vi "XY Graph Add Single Plot with Name v2.vi"(0 "XYGraph Ref in":T3, 1 "Scales (Default)":T2, 3 "Keep Existing Plots (T)":bool=TRUE, 5 "Plot":cluster{"X Array":dbl[], "Y Array":dbl[]}, 7 "Plot Metadata":variant, 9 "Plot Name (\"Plot\")":string, 11 "error in (no error)":errorcluster, 12 "Plot Style":T1) -> (4 "XY Graph Caption (or Label)":string, 8 "Plot Index":i32, 10 "Plot Name":string, 15 "error out":errorcluster)   [LabVIEW 2021, in "XY Graph Add-Ons.lvlib"]
uses:
  XY Graph Add-Ons.lvlib
  XY Graph Refnum.ctl
  Plot Scales.ctl
  Single Plot Style 2.ctl
  XY Graph Get Plots Metadata.vi
  XY Graph Get Max Legend Size.vi
  XY Graph Set Plots Metadata.vi
  Strings/Strings.lvlib
  Graphs.lvlib
  Error/Error.lvlib
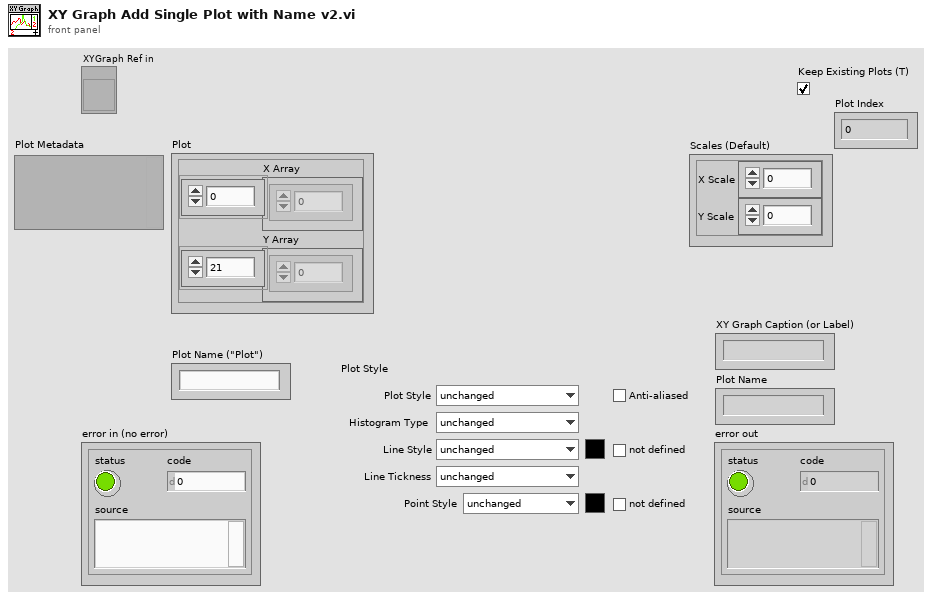
[diagram p1: front panel]
types:
  T1 = typedef "Graphs.lvlib/Single Plot Style 2.ctl" = cluster{"Plot Style":enum16{"unchanged", "Line", "Symbol", "Line + Symbol", "Histogram", "Histogram + Symbol"}, "Histogram Type":enum16{"unchanged", "Left Bound", "Center", "Right Bound"}, "Line Tickness":enum16{"unchanged", "Thin", "1 pixel", "2 pixel", "3 pixel", "4 pixel", "5 pixel"}, "Line Style":enum16{"unchanged", "Plain", "Long Dash", "Short Dash", "Long-Short Dash", "Long-Short-Short Dash"}, "Point Style":enum16{"unchanged", "None", "Empty Circle", "Filled Circle", "Thick Circle", "Dotted Circle", "Empty Square", "Filled Square", "Thick Square", "Dotted Square", "Small Filled Square", "Dot", "Cross", "Tiny Cross", "Large X", "Small x", "Diamond", "Small Empty Square"}, "Line Color":u32, "Line Color defined?":bool, "Point Color":u32, "Point Color defined?":bool, "Anti-aliased":bool}
  T2 = typedef "XY Graph Add-Ons.lvlib/Plot Scales.ctl" = cluster{"X Scale":u32, "Y Scale":u32}
  T3 = typedef "XY Graph Add-Ons.lvlib/XY Graph Refnum.ctl" = refnum<vi>
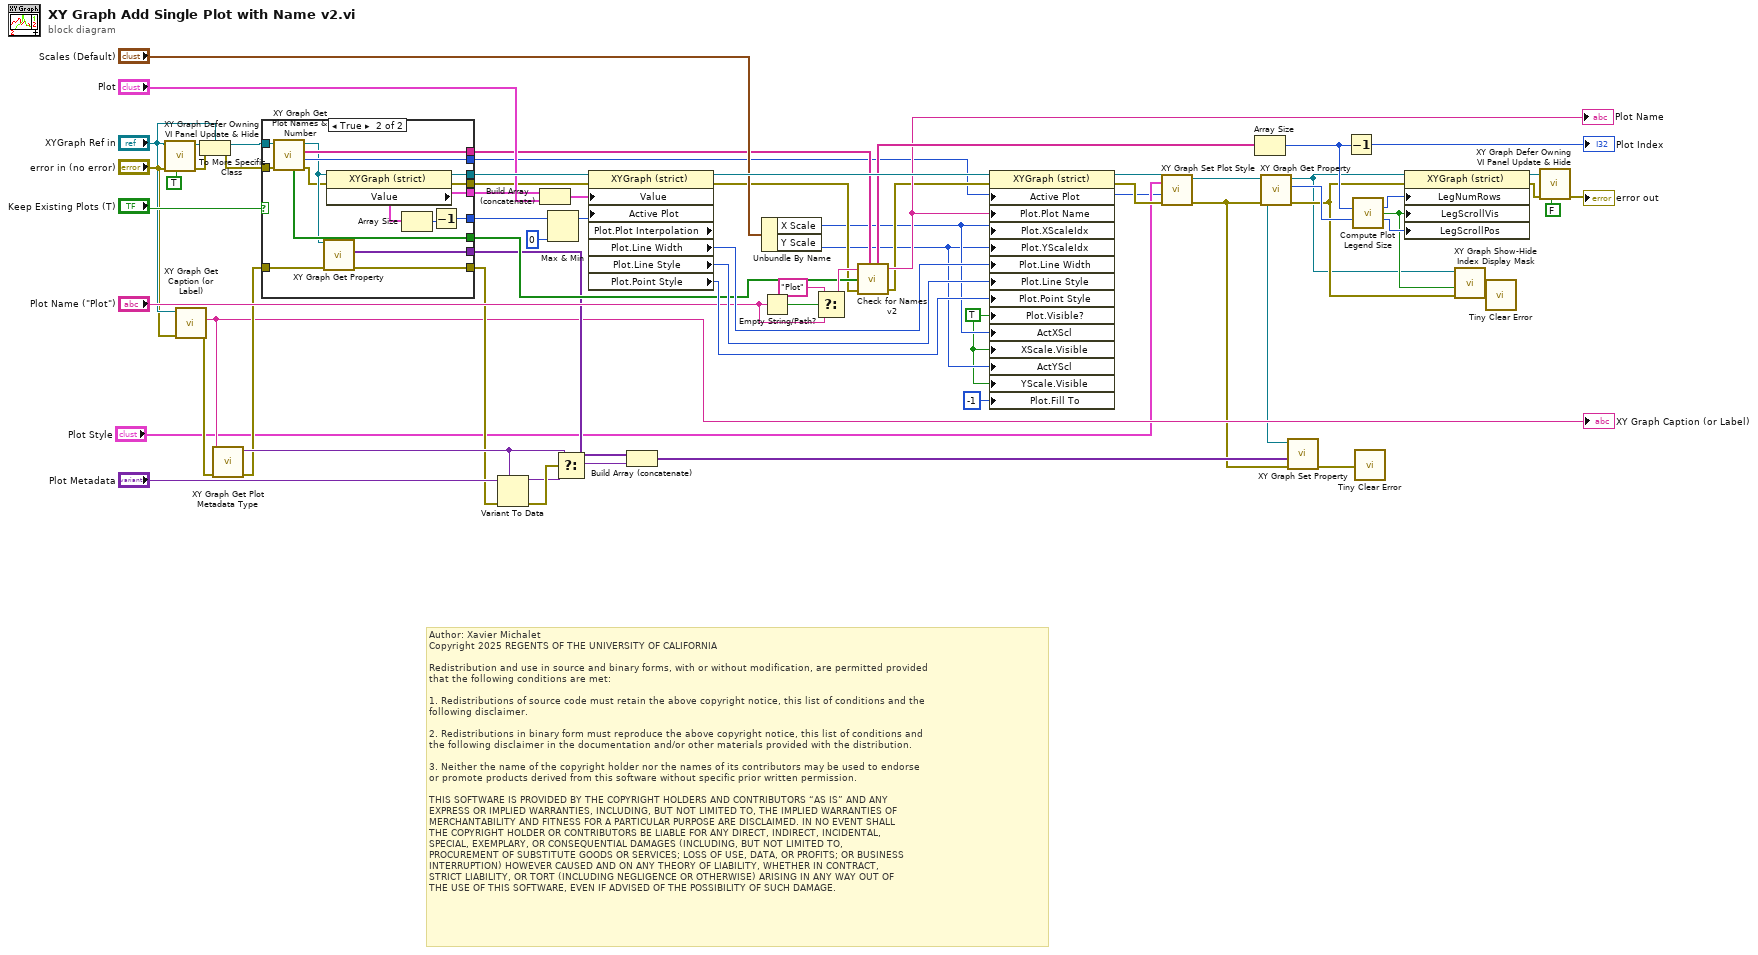
[diagram p0: block diagram]
diagram:
  w8 = TRUE ("Plot.Visible")
  # "Author: Xavier Michalet\nCopyright 2025 REGENTS OF THE UNIVERSITY OF CALIFORNIA\n\nRedistribution and use in source and binary forms, with or without modification, are permitted provided\nthat the following conditions are met:\n\n1. Redistributions of source code must retain the above copyright notice, this list of conditions and the\nfollowing disclaimer.\n\n2. Redistributions in binary form must reproduce the above copyright notice, this list of conditions and\nthe following disclaimer in the documentation and/or other materials provided with the distribution.\n\n3. Neither the name of the copyright holder nor the names of its contributors may be used to endorse \nor promote products derived from this software without specific prior written permission.\n\nTHIS SOFTWARE IS PROVIDED BY THE COPYRIGHT HOLDERS AND CONTRIBUTORS “AS IS” AND ANY \nEXPRESS OR IMPLIED WARRANTIES, INCLUDING, BUT NOT LIMITED TO, THE IMPLIED WARRANTIES OF\nMERCHANTABILITY AND FITNESS FOR A PARTICULAR PURPOSE ARE DISCLAIMED. IN NO EVENT SHALL\nTHE COPYRIGHT HOLDER OR CONTRIBUTORS BE LIABLE FOR ANY DIRECT, INDIRECT, INCIDENTAL, \nSPECIAL, EXEMPLARY, OR CONSEQUENTIAL DAMAGES (INCLUDING, BUT NOT LIMITED TO, \nPROCUREMENT OF SUBSTITUTE GOODS OR SERVICES; LOSS OF USE, DATA, OR PROFITS; OR BUSINESS\nINTERRUPTION) HOWEVER CAUSED AND ON ANY THEORY OF LIABILITY, WHETHER IN CONTRACT, \nSTRICT LIABILITY, OR TORT (INCLUDING NEGLIGENCE OR OTHERWISE) ARISING IN ANY WAY OUT OF\nTHE USE OF THIS SOFTWARE, EVEN IF ADVISED OF THE POSSIBILITY OF SUCH DAMAGE."
  n1 = call "XY Graph Defer Owning VI Panel Update & Hide.vi"("Defer Owning Panel Update"=TRUE, "error in (no error)"="error in (no error)", "XY Graph Refnum in"="XYGraph Ref in") -> ("error out"=w37:errorcluster, "XY Graph Refnum out"=w44:refnum<vi>)  [unwired: 7 in]
  n2 = call "XY Graph Get Caption (or Label).vi"("error in (no error)"="error in (no error)", "XY Graph in"="XYGraph Ref in") -> ("error out"=w16:errorcluster, "Caption (or Label) Text"=w15:string)  [unwired: 7 in, 1 out]
  "XY Graph Caption (or Label)" <- w15
  n3 = To More Specific Class(target class="XYGraph Ref in", reference=w44, error in=w37) -> (specific class reference=w38:T3, error out=w36:errorcluster)
  n4 = call "XY Graph Get Plot Metadata Type.vi"("Error In"=w16, "Graph Label"=w15) -> ("Error Out"=w19:errorcluster, "Plot Metadata Type"=w22:variant)  [unwired: 7 in, 1 out]
  n5 = case shown="True" "Keep Existing Plots (T)" {
    tunnel: w38 -> [w69 w84]
    tunnel: [w69 w83] -> w65
    tunnel: w36 -> [w68 w82]
    tunnel: [_ w81] -> w62
    tunnel: [_ w79] -> w61
    tunnel: [_ w78] -> w49
    tunnel: [_ w77] -> w4
    tunnel: [w68 w76] -> w51
    tunnel: [_ w75] -> w41
    tunnel: [_ w72] -> w28
    tunnel: w19 -> [w67 w71]
    tunnel: [w67 w70] -> w18
    frame False {
    }
    frame True {
      n6 = call "XY Graph Get Plot Names & Number.vi"("error in (no error)"=w82, "XYGraph in"=w84) -> ("error out"=w73:errorcluster, "# Plots"=w77:i32, "Plot Names"=w78:string[], "XYGraph out"=w74:T3, "Empty Plots?"=w75:bool[])  [unwired: 4 in, 1 out]
      n7 = call-poly "XY Graph Get Property.vi"("Error In"=w71, "XYGraph Ref"=w74) -> ("Error Out"=w70:errorcluster, "Plot Metadata"=w72:variant[])  [unwired: 6 in, 2 out]
      n8 = property class="XYGraph (strict)"(reference=w74, error in=w73) -> (reference out=w83:T3, error out=w76:errorcluster, "Value"=w81:cluster{"X Array":dbl[], "Y Array":dbl[]}[])
      n9 = Array Size(array=w81) -> (size(s)=w80:i32)
      n10 = Decrement(x=w80) -> (x-1=w79:i32)
    }
  }
  n11 = Variant To Data(error in=w18, type=w22, Variant="Plot Metadata") -> (data=w21:variant, error out=w23:errorcluster)
  n12 = Build Array (concatenate)(w62, "Plot") -> (w66:cluster{"X Array":dbl[], "Y Array":dbl[]}[])
  n13 = Max & Min(x=w61, y=0) -> (max(x,y)=w53:i32)  [unwired: 1 out]
  n14 = Select(t=w22, s=w23, f=w21) -> (s? t:f=w20:variant)
  n15 = property class="XYGraph (strict)" props=["Value", "Active Plot", "Plot", "Plot Interpolation", "Plot", "Line Width", "Plot", "Line Style", "Plot", "Point Style"](reference=w65, error in=w51, "Value"=w66, "Active Plot"=w53) -> (reference out=w64:T3, error out=w40:errorcluster, "Plot.Line Width"=w60:u8, "Plot.Line Style"=w59:u8, "Plot.Point Style"=w58:u8)  [unwired: 1 out]
  n16 = Build Array (concatenate)(w28, w20) -> (w27:variant[])
  n17 = Unbundle By Name("Scales (Default)") -> ("X Scale"=w10:u32, "Y Scale"=w9:u32)
  n18 = Empty String/Path?(string/path="Plot Name (\"Plot\")") -> (empty?=w57:bool)
  n19 = Select(t="Plot", s=w57, f="Plot Name (\"Plot\")") -> (s? t:f=w47:string)
  n20 = call "Check for Names v2.vi"("New Name"=w47, "Name List"=w49, "Empty Plots?"=w41, "Error In"=w40) -> ("New Name List"=w48:string[], "New Name"=w46:string, "Error Out"=w39:errorcluster)  [unwired: 2 in, 1 out]
  "Plot Name" <- w46
  n21 = property class="XYGraph (strict)"(reference=w64, error in=w39, "Active Plot"=w4, "Plot.Plot Name"=w46, "Plot.XScaleIdx"=w10, "Plot.YScaleIdx"=w9, "Plot.Line Width"=w60, "Plot.Line Style"=w59, "Plot.Point Style"=w58, "Plot.Visible?"=w8, "ActXScl"=w10, "XScale.Visible"=w8, "ActYScl"=w9, "YScale.Visible"=w8, "Plot.Fill To"=i16 -1) -> (reference out=w7:T3, error out=w6:errorcluster)
  n22 = call "XY Graph Set Plot Style.vi"("Error In"=w6, "Plot Index (0)"=w4, "Single Plot Style"="Plot Style", "XY Graph Refnum in"=w7) -> ("Error Out"=w2:errorcluster, "XY Graph Refnum out"=w3:T3)  [unwired: 6 in]
  n23 = Array Size(array=w48) -> (size(s)=w34:i32)
  n24 = call-poly "XY Graph Get Property.vi"("Error In"=w2, "XYGraph Refnum"=w3) -> ("Error Out"=w12:errorcluster, "Max Legend Size"=w35:i32, "XYGraph Refnum"=w11:T3)  [unwired: 6 in, 1 out]
  n25 = call-poly "XY Graph Set Property.vi"("error in (no error)"=w2, "Plots Metadata"=w27, "XY Graph Refnum"=w3) -> ("error out"=w26:errorcluster)  [unwired: 7 in, 1 out]
  n26 = Decrement(x=w34) -> (x-1=→"Plot Index":i32)
  n27 = call "Compute Plot Legend Size.vi"("# Plots"=w34, "Max Legend Size"=w35) -> ("LegNumRows"=w33:u32, "LegScrollVis"=w13:bool, "LegScrollPos"=w32:u32)  [unwired: 11 in]
  n28 = call "Tiny Clear Error.vi"("Error In"=w26) -> ()  [unwired: 8 in, 1 out]
  n29 = property class="XYGraph (strict)"(reference=w11, error in=w12, "LegNumRows"=w33, "LegScrollVis"=w13, "LegScrollPos"=w32) -> (reference out=w29:T3, error out=w42:errorcluster)
  n30 = call "XY Graph Show-Hide Index Display Mask.vi"("error in (no error)"=w12, "Show(T)/Hide(F)"=w13, "XYGraph Ref"=w11) -> ("error out"=w14:errorcluster)  [unwired: 7 in, 1 out]
  n31 = call "Tiny Clear Error.vi"("Error In"=w14) -> ()  [unwired: 8 in, 1 out]
  n32 = call "XY Graph Defer Owning VI Panel Update & Hide.vi"("Defer Owning Panel Update"=FALSE, "error in (no error)"=w42, "XY Graph Refnum in"=w29) -> ("error out"=→"error out":errorcluster)  [unwired: 7 in, 1 out]
